vi "ACC_LabVIEW_Write.vi"(0 "DeviceReferenceIn":cluster{"ID":u32}, 2 "Propname":string, 3 "Acc_Para_In":T1[](array[typedef]), 4 "Acc_Data_In":T1[](array[typedef])=[{"Data Type"=enum."UWord (16Bit Int unsigned)", "String"="", "Double"=1.0}], 5 "error in (no error)":errorcluster, 7 "Error strings buffer size (Byte)":u32=500, 8 "VirtAcc":i32) -> (14 "DeviceReferenceOut":cluster{"ID":u32}, 17 "Acc_Data_Out":T1[](array[typedef]), 19 "error out":errorcluster)   [LabVIEW 2014, in "ACC_LabVIEW.lvlib"]
doc: "Perform a \"write\" inside the GSI - accelerator control system."
uses:
  ACC_LabVIEW.lvlib
  lib/ACC_Interface_Wrapper.dll
  ACC_LabVIEW_DataTypes.ctl
  ACC_LabVIEW_Container.ctl
panel:
  in  "AccData Container":T1={"Data Type"=enum."UByte (8Bit int unsigned)", "String"="", "Double"=0.0}
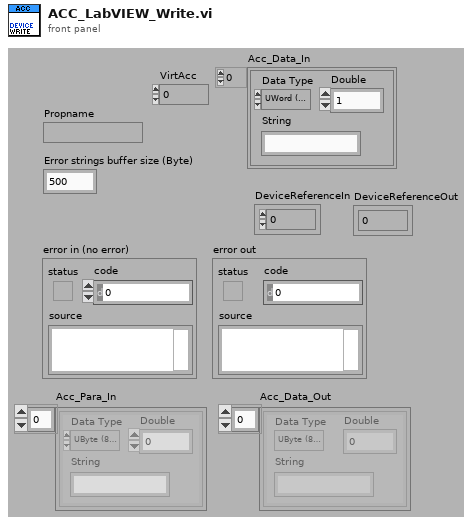
[diagram p1: front panel]
types:
  T1 = typedef "ACC_LabVIEW.lvlib/ACC_LabVIEW_Container.ctl" = cluster{"Data Type":T2, "String":string, "Double":dbl}
  T2 = typedef "ACC_LabVIEW.lvlib/ACC_LabVIEW_DataTypes.ctl" = enum16{"SByte (8Bit Int signed)", "UByte (8Bit int unsigned)", "SWord (16Bit Int signed)", "UWord (16Bit Int unsigned)", "SLong (32Bit Int signed)", "ULong (32Bit Int unsigned)", "Float32 (float)", "Float64 (double)", "String"}
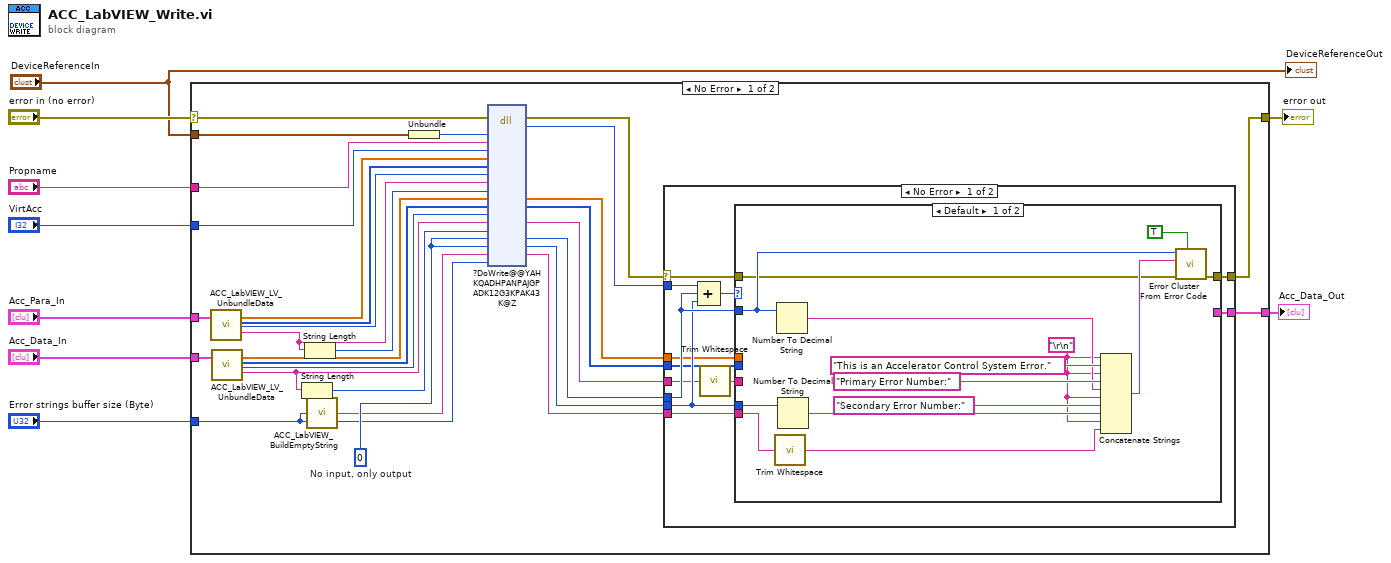
[diagram p0: block diagram]
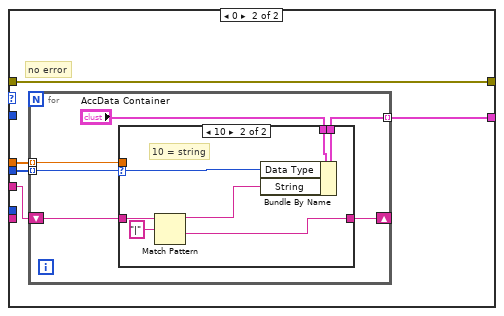
[diagram p2: hidden frame]
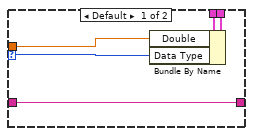
[diagram p3: hidden frame]
diagram:
  n1 = case shown="No Error" "error in (no error)" {
    selector: "error in (no error)" -> [w35 w90]
    tunnel: "Propname" -> [w34 _]
    tunnel: "VirtAcc" -> [w33 _]
    tunnel: [w39 w90] -> w7
    tunnel: [w38 _] -> w6
    tunnel: "Error strings buffer size (Byte)" -> [w20 _]
    tunnel: "Acc_Para_In" -> [w37 _]
    tunnel: "Acc_Data_In" -> [w36 _]
    tunnel: "DeviceReferenceIn" -> [w11 _]
    frame No Error {
      w22 = u32 0  # No input, only output
      n2 = call "ACC_LabVIEW_LV_UnbundleData.vi"("Acc_Data_In"=w37) -> ("LV_double_array"=w32:dbl[], "LV_types"=w31:i32[], "Length"=w30:i32, "Data-String"=w29:string)  [unwired: 15 in]
      n3 = call "ACC_LabVIEW_LV_UnbundleData.vi"("Acc_Data_In"=w36) -> ("LV_double_array"=w27:dbl[], "LV_types"=w26:i32[], "Length"=w25:i32, "Data-String"=w24:string)  [unwired: 15 in]
      n4 = String Length(string=w24) -> (length=w23:i32)
      n5 = String Length(string=w29) -> (length=w28:i32)
      n6 = call "ACC_LabVIEW_BuildEmptyString.vi"("Length"=w20) -> ("String"=w21:string)
      n7 = Unbundle(w11) -> ("ID"=w10:u32)
      n8 = dll-call lib="D:/Git/CS-framework/instr.lib/ACC_LabVIEW_Interface/lib/ACC_Interface_Wrapper.dll" fn="?DoWrite@@YAHKQADHPANPAJGPADK12G3KPAK43K@Z"(error in=w35, "DeviceHandle"=w10, "LV_propname"=w34, "LV_VirtAcc"=w33, "LV_para"=w32, "LV_para_types"=w31, "LV_para_Size"=w30, "LV_para_string"=w29, "LV_para_string_Size"=w28, "LV_data"=w27, "LV_data_types"=w26, "LV_data_Size"=w25, "LV_data_string"=w24, "LV_data_string_Size"=w23, "ErrPrimStat"=w22, "ErrSecStat"=w22, "ErrorMSG"=w21, "ErrorMSG_Size"=w20) -> (error out=w19:errorcluster, "return type"=w18:i32, "LV_data"=w17:dbl[], "LV_data_types"=w16:i32[], "LV_data_string"=w15:string, "ErrPrimStat"=w14:u32, "ErrSecStat"=w13:u32, "ErrorMSG"=w12:string)  [unwired: 13 in, 1 out]
      n9 = case shown="No Error" w19 {
        selector: w19 -> [w49 w89]
        tunnel: w18 -> [w51 _]
        tunnel: [w46 w89] -> w39
        tunnel: w12 -> [w40 _]
        tunnel: w14 -> [w48 _]
        tunnel: w13 -> [w47 _]
        tunnel: w17 -> [w45 _]
        tunnel: w16 -> [w44 _]
        tunnel: w15 -> [w41 _]
        tunnel: [w43 _] -> w38
        frame No Error {
          n10 = Compound Arithmetic op=ADD(w51, w48, w47) -> (w50:u32)
          n11 = call <vilib>:"Trim Whitespace.vi"("string"=w41) -> ("trimmed string"=w42:string)  [unwired: 1 in]
          n12 = case shown="Default" w50 {
            tunnel: w42 -> [_ w67]
            tunnel: w49 -> [w54 w70]
            tunnel: w48 -> [w55 _]
            tunnel: w47 -> [w65 _]
            tunnel: [w53 w70] -> w46
            tunnel: w45 -> [_ w69]
            tunnel: w44 -> [_ w68]
            tunnel: [_ w66] -> w43
            tunnel: w40 -> [w59 _]
            frame Default {
              w58 = "\r\n"
              n13 = call <vilib>:"Trim Whitespace.vi"("string"=w59) -> ("trimmed string"=w57:string)  [unwired: 1 in]
              n14 = Number To Decimal String(number=w55) -> (decimal integer string=w62:string)  [unwired: 1 in]
              n15 = Number To Decimal String(number=w65) -> (decimal integer string=w60:string)  [unwired: 1 in]
              n16 = Concatenate Strings(w58, "This is an Accelerator Control System Error.", w58, "Primary Error Number:", w62, w58, "Secondary Error Number:", w60, w58, w57) -> (w56:string)
              n17 = call <vilib>:"Error Cluster From Error Code.vi"("show call chain? (False)"=TRUE, "error in (no error)"=w54, "error message (\"\")"=w56, "error code (0)"=w55) -> ("error out"=w53:errorcluster)  [unwired: 5 in]
            }
            frame 0 {
              # "no error"
              n18 = for {
                tunnel: w69 -> [w75] mode=indexing
                tunnel: w68 -> [w74] mode=indexing
                shift-right: [w72] -> _
                shift-left: w67 -> [w73]
                tunnel: [w71] -> w66 mode=indexing
                n19 = case shown="10" w74 {
                  selector: w74 -> [w79 w87]
                  tunnel: "AccData Container" -> [w78 w88]
                  tunnel: w75 -> [w81 _]
                  tunnel: w73 -> [w80 w86]
                  tunnel: [w80 w84] -> w72
                  tunnel: [w77 w82] -> w71
                  frame Default {
                    n20 = Bundle By Name(cluster=w78, "Double"=w81, "Data Type"=w79) -> (w77:T1)
                  }
                  frame 10 {
                    # "10 = string"
                    n21 = Match Pattern(string=w86, regular expression="|") -> (before substring=w83:string, after substring=w84:string)  [unwired: 1 in, 2 out]
                    n22 = Bundle By Name(cluster=w88, "Data Type"=w87, "String"=w83) -> (w82:T1)
                  }
                }
              }
            }
          }
        }
        frame Error {
        }
      }
    }
    frame Error {
    }
  }
  "error out" <- w7
  "Acc_Data_Out" <- w6
  "DeviceReferenceOut" <- "DeviceReferenceIn"
